vi "Measurement Logic.vi"() -> ()   [LabVIEW 2021, in "PSRR_PMIC.lvlib"]
uses:
  PSRR_PMIC.lvlib
  Measurement Results.ctl
  <instrlib>/niDCPower/nidcpower.llb/niDCPower Get Channel Name From String.vi
  <instrlib>/niDCPower/nidcpower.llb/niDCPower Source Mode.ctl
  <instrlib>/niDCPower/nidcpower.llb/niDCPower Output Function.ctl
  <instrlib>/niDCPower/nidcpower.llb/niDCPower Sense.ctl
  <instrlib>/niDCPower/nidcpower.llb/niDCPower Wait For Event - Event.ctl
  <instrlib>/niFgen/niFgen.llb/niFgen Output Mode.ctl
  <instrlib>/niScope/Controls/niScope vertical coupling.ctl
  <instrlib>/niScope/Controls/niScope trigger slope.ctl
  <instrlib>/niScope/Controls/niScope trigger coupling.ctl
  <instrlib>/niScope/Controls/niScope trigger source.ctl
  <instrlib>/niScope/Utility/niScope Get Channel Name From String.vi
  <instrlib>/niScope/Configure/Trigger/niScope Configure Trigger Edge.vi
  <vilib>/Plug-In SDKs/Measurements/Measure Call Context/Measure Call Context.lvclass
  Measurement Configuration.ctl
panel:
  out "measurement results":T1
  in  "measurement configuration":T2={"DUT setup time"=1.0, "Source resource name"="", "Source current limit"=0.15, "Source voltage level"=10.0, "Load resource name"="", "Load voltage limit range"=6.0, "Load current level"=0.025, "Fgen resource name"="", "Fgen channel name"="", "Fgen pk-pk amplitude"=1.0, "Fgen load impedance"=10000.0, "Fgen start frequency"=10.0, "Fgen stop frequency"=10000000.0, "Fgen frequency sweep points/points per decade"=10, "Fgen sweep type"="Logarithmic", "Fgen standard Waveform"=enum."Sine", "Scope resource name"="", "Scope input channel name"="", "Scope output channel name"="", "Scope probe attenuation"=1.0, "Scope samples per cycle"=1000, "Scope cycles to average"=4} {"Fgen start frequency" format="%#_6p"; "Fgen load impedance" format="%#_6p"; "Fgen pk-pk amplitude" format="%#_6p"}
  out "measure call context out":refnum<class "Measure Call Context.lvclass">
  in  "measure call context in":refnum<class "Measure Call Context.lvclass">
  out "error out":errorcluster
  in  "error in":errorcluster
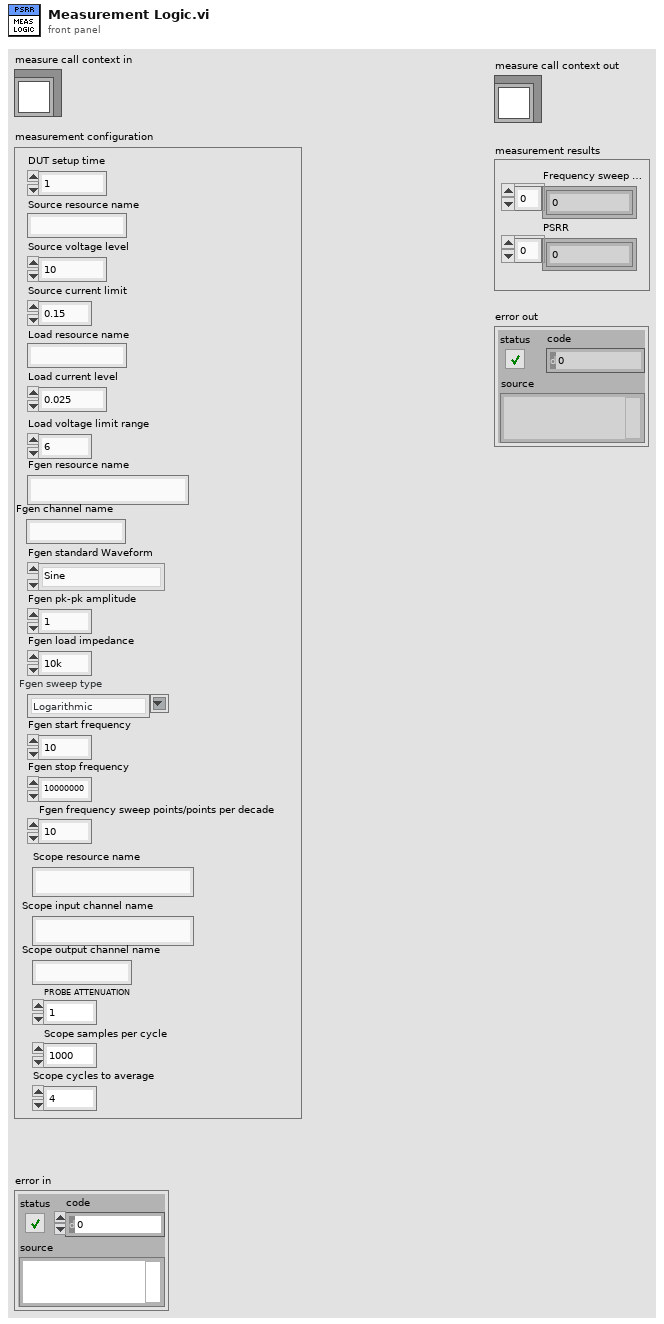
[diagram p1: front panel]
types:
  T1 = typedef "PSRR_PMIC.lvlib/Measurement Results.ctl" = cluster{"Frequency sweep points":dbl[], "PSRR":dbl[]}
  T2 = typedef "PSRR_PMIC.lvlib/Measurement Configuration.ctl" = cluster{"DUT setup time":dbl, "Source resource name":string, "Source current limit":dbl, "Source voltage level":dbl, "Load resource name":string, "Load voltage limit range":dbl, "Load current level":dbl, "Fgen resource name":string, "Fgen channel name":string, "Fgen pk-pk amplitude":dbl, "Fgen load impedance":dbl, "Fgen start frequency":dbl, "Fgen stop frequency":dbl, "Fgen frequency sweep points/points per decade":i32, "Fgen sweep type":string, "Fgen standard Waveform":enum32{"Sine", "Square", "Triangle", "Ramp Up", "Ramp Down", "DC", "Noise"}, "Scope resource name":string, "Scope input channel name":string, "Scope output channel name":string, "Scope probe attenuation":dbl, "Scope samples per cycle":i32, "Scope cycles to average":i32}
  T3 = typedef "niScope trigger coupling.ctl" = u16
  T4 = typedef "niScope trigger slope.ctl" = i32
  T5 = typedef "niScope vertical coupling.ctl" = i32
  T6 = typedef "niFgen Output Mode.ctl" = u32
  T7 = typedef "niDCPower Output Function.ctl" = i32
  T8 = typedef "niDCPower Source Mode.ctl" = i32
  T9 = typedef "niDCPower Wait For Event - Event.ctl" = i32
  T10 = typedef "niDCPower Sense.ctl" = i32
  T11 = enum32{"Sine", "Square", "Triangle", "Ramp Up", "Ramp Down", "DC", "Noise"}
  T12 = typedef "niScope trigger source.ctl" = string
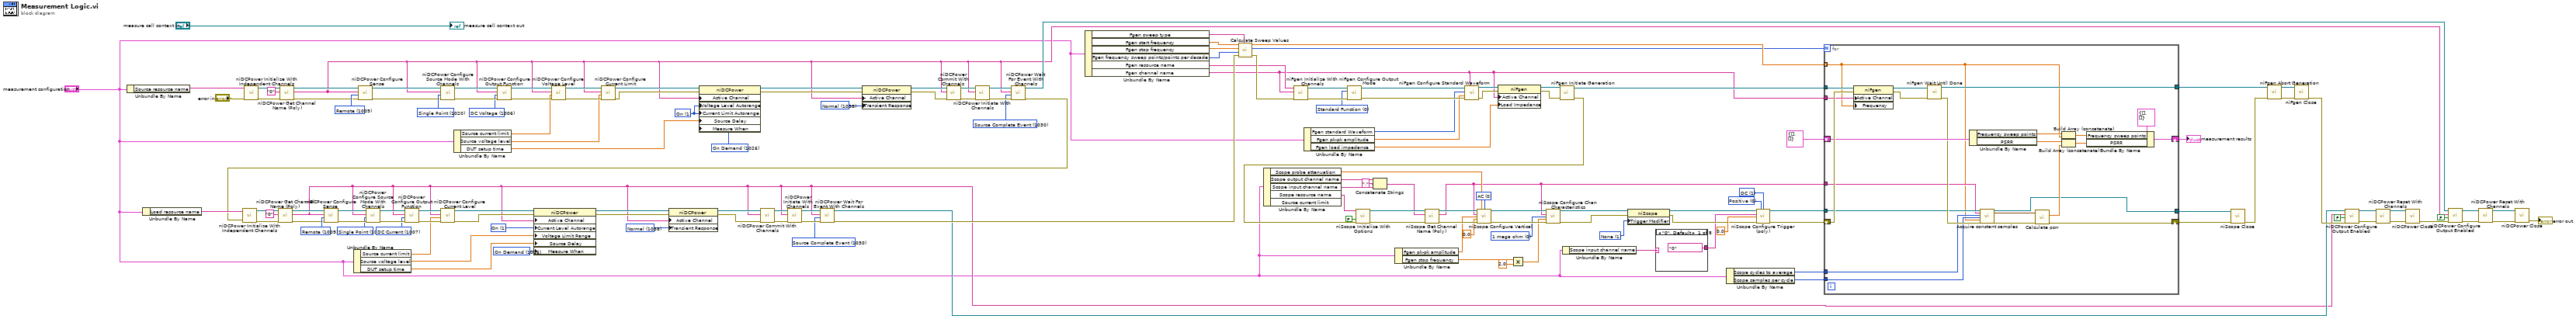
[diagram p0: block diagram]
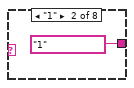
[diagram p2: hidden frame]
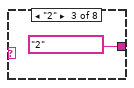
[diagram p3: hidden frame]
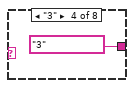
[diagram p4: hidden frame]
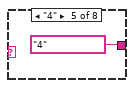
[diagram p5: hidden frame]
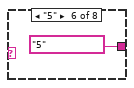
[diagram p6: hidden frame]
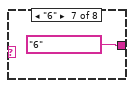
[diagram p7: hidden frame]
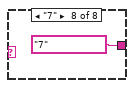
[diagram p8: hidden frame]
diagram:
  w51 = 1 items=["None"=1, "Auto Trigger"=2] ("Triggering:Trigger Modifier")
  w57 = T3 1 items=["AC"=0, "DC"=1, "HF Reject"=3, "LF Reject"=4, "AC Plus HF Reject"=1001] ("trigger coupling")
  w58 = T4 0 items=["Positive", "Negative"] ("trigger slope")
  w60 = T5 0 items=["AC", "DC", "Ground"] ("vertical coupling")
  w63 = u32 0 items=["1 mega ohm"=0, "50 ohms"=2] ("input impedance")
  w79 = T6 0 items=["Standard Function", "Frequency List", "Arbitrary Waveform", "Arbitrary Sequence", "Script"] ("Output Mode (default: 0=Standard Function)")
  w98 = T7 1007 items=["DC Voltage"=1006, "DC Current"=1007, "Pulse Voltage"=1049, "Pulse Current"=1050] ("output function")
  w99 = T8 1020 items=["Single Point"=1020, "Sequence"=1021] ("source mode")
  w24 = 1026 items=["Automatically after Source Complete"=1025, "On Demand"=1026, "On Measure Trigger"=1027] ("Measurement:Advanced:Measure When")
  w101 = 1 items=["Off", "On"] ("Source:DC Current:Current Level Autorange")
  w113 = 1038 items=["Slow"=1041, "Normal"=1038, "Fast"=1039, "Custom"=1042] ("Source:Transient Response")
  w116 = T9 1030 items=["Source Complete Event"=1030, "Measure Complete Event"=1031, "Sequence Iteration Complete Event"=1032, "Sequence Engine Done Event"=1033, "Pulse Complete Event"=1051, "Ready For Pulse Trigger Event"=1052] ("event")
  w119 = T10 1009 items=["Local"=1008, "Remote"=1009] ("sense")
  w122 = T9 1030 items=["Source Complete Event"=1030, "Measure Complete Event"=1031, "Sequence Iteration Complete Event"=1032, "Sequence Engine Done Event"=1033, "Pulse Complete Event"=1051, "Ready For Pulse Trigger Event"=1052] ("event")
  w130 = 1038 items=["Slow"=1041, "Normal"=1038, "Fast"=1039, "Custom"=1042] ("Source:Transient Response")
  w137 = T10 1009 items=["Local"=1008, "Remote"=1009] ("sense")
  w138 = 1026 items=["Automatically after Source Complete"=1025, "On Demand"=1026, "On Measure Trigger"=1027] ("Measurement:Advanced:Measure When")
  w144 = 1 items=["Off", "On"] ("Source:DC Voltage:Current Limit Autorange")
  w146 = T7 1006 items=["DC Voltage"=1006, "DC Current"=1007, "Pulse Voltage"=1049, "Pulse Current"=1050] ("output function")
  w149 = T8 1020 items=["Single Point"=1020, "Sequence"=1021] ("source mode")
  n1 = Unbundle By Name("measurement configuration") -> ("Source resource name"=w150:string)
  n2 = Unbundle By Name("measurement configuration") -> ("Load resource name"=w89:string)
  n3 = call <instrlib>:"niDCPower Initialize With Independent Channels.vi"("error in (no error)"="error in", "resource name"=w150) -> ("error out"=w152:errorcluster, "instrument handle out"=w153:refnum<k15>)  [unwired: 8 in]
  n4 = call-poly <instrlib>:"niDCPower Get Channel Name (Poly).vi"("error in (no error)"=w152, "index"="0", "instrument handle"=w153) -> ("error out"=w120:errorcluster, "name"=w8:string, "instrument handle out"=w121:refnum<k15>)  [unwired: 6 in]
  n5 = Unbundle By Name("measurement configuration") -> ("Source current limit"=w100:dbl, "Source voltage level"=w95:dbl, "DUT setup time"=w110:dbl)
  n6 = call <instrlib>:"niDCPower Configure Sense.vi"("error in (no error)"=w120, "sense"=w137, "channel name"=w8, "instrument handle"=w121) -> ("error out"=w129:errorcluster, "instrument handle out"=w128:refnum<k15>)  [unwired: 6 in]
  n7 = call <instrlib>:"niDCPower Configure Source Mode With Channels.vi"("error in (no error)"=w129, "source mode"=w149, "channel name"=w8, "instrument handle"=w128) -> ("error out"=w148:errorcluster, "instrument handle out"=w147:refnum<k15>)  [unwired: 6 in]
  n8 = Unbundle By Name("measurement configuration") -> ("Source current limit"=w126:dbl, "Source voltage level"=w127:dbl, "DUT setup time"=w125:dbl)
  n9 = call <instrlib>:"niDCPower Configure Output Function.vi"("error in (no error)"=w148, "output function"=w146, "channel name"=w8, "instrument handle"=w147) -> ("error out"=w142:errorcluster, "instrument handle out"=w141:refnum<k15>)  [unwired: 6 in]
  n10 = call <instrlib>:"niDCPower Configure Voltage Level.vi"("error in (no error)"=w142, "voltage level"=w126, "channel name"=w8, "instrument handle"=w141) -> ("error out"=w139:errorcluster, "instrument handle out"=w140:refnum<k15>)  [unwired: 6 in]
  n11 = call <instrlib>:"niDCPower Configure Current Limit.vi"("error in (no error)"=w139, "current limit"=w127, "channel name"=w8, "instrument handle"=w140) -> ("error out"=w145:errorcluster, "instrument handle out"=w143:refnum<k15>)  [unwired: 6 in]
  n12 = property class="niDCPower"(reference=w143, error in=w145, "Active Channel"=w8, "Voltage Level Autorange"=w144, "Current Limit Autorange"=w144, "Source Delay"=w125, "Measure When"=w138) -> (reference out=w134:refnum<k15>, error out=w133:errorcluster)
  n13 = property class="niDCPower"(reference=w134, error in=w133, "Active Channel"=w8, "Transient Response"=w130) -> (reference out=w132:refnum<k15>, error out=w131:errorcluster)
  n14 = call <instrlib>:"niDCPower Commit With Channels.vi"("error in (no error)"=w131, "channel name"=w8, "instrument handle"=w132) -> ("error out"=w135:errorcluster, "instrument handle out"=w136:refnum<k15>)  [unwired: 7 in]
  n15 = call <instrlib>:"niDCPower Initiate With Channels.vi"("error in (no error)"=w135, "channel name"=w8, "instrument handle"=w136) -> ("error out"=w123:errorcluster, "instrument handle out"=w124:refnum<k15>)  [unwired: 7 in]
  n16 = call <instrlib>:"niDCPower Wait For Event With Channels.vi"("error in (no error)"=w123, "event"=w122, "channel name"=w8, "instrument handle"=w124) -> ("error out"=w70:errorcluster, "instrument handle out"=w11:refnum<k15>)  [unwired: 6 in]
  n17 = call <instrlib>:"niDCPower Initialize With Independent Channels.vi"("error in (no error)"=w70, "resource name"=w89) -> ("error out"=w93:errorcluster, "instrument handle out"=w94:refnum<k15>)  [unwired: 8 in]
  n18 = call-poly <instrlib>:"niDCPower Get Channel Name (Poly).vi"("error in (no error)"=w93, "index"="0", "instrument handle"=w94) -> ("error out"=w90:errorcluster, "name"=w9:string, "instrument handle out"=w91:refnum<k15>)  [unwired: 6 in]
  n19 = call <instrlib>:"niDCPower Configure Sense.vi"("error in (no error)"=w90, "sense"=w119, "channel name"=w9, "instrument handle"=w91) -> ("error out"=w104:errorcluster, "instrument handle out"=w107:refnum<k15>)  [unwired: 6 in]
  n20 = call <instrlib>:"niDCPower Configure Source Mode With Channels.vi"("error in (no error)"=w104, "source mode"=w99, "channel name"=w9, "instrument handle"=w107) -> ("error out"=w103:errorcluster, "instrument handle out"=w106:refnum<k15>)  [unwired: 6 in]
  n21 = call <instrlib>:"niDCPower Configure Output Function.vi"("error in (no error)"=w103, "output function"=w98, "channel name"=w9, "instrument handle"=w106) -> ("error out"=w102:errorcluster, "instrument handle out"=w105:refnum<k15>)  [unwired: 6 in]
  n22 = call <instrlib>:"niDCPower Configure Current Level.vi"("error in (no error)"=w102, "current level"=w100, "channel name"=w9, "instrument handle"=w105) -> ("error out"=w96:errorcluster, "instrument handle out"=w97:refnum<k15>)  [unwired: 6 in]
  n23 = property class="niDCPower"(reference=w97, error in=w96, "Active Channel"=w9, "Current Level Autorange"=w101, "Voltage Limit Range"=w95, "Source Delay"=w110, "Measure When"=w24) -> (reference out=w112:refnum<k15>, error out=w111:errorcluster)
  n24 = property class="niDCPower"(reference=w112, error in=w111, "Active Channel"=w9, "Transient Response"=w113) -> (reference out=w109:refnum<k15>, error out=w108:errorcluster)
  n25 = call <instrlib>:"niDCPower Commit With Channels.vi"("error in (no error)"=w108, "channel name"=w9, "instrument handle"=w109) -> ("error out"=w114:errorcluster, "instrument handle out"=w115:refnum<k15>)  [unwired: 7 in]
  n26 = call <instrlib>:"niDCPower Initiate With Channels.vi"("error in (no error)"=w114, "channel name"=w9, "instrument handle"=w115) -> ("error out"=w118:errorcluster, "instrument handle out"=w117:refnum<k15>)  [unwired: 7 in]
  n27 = call <instrlib>:"niDCPower Wait For Event With Channels.vi"("error in (no error)"=w118, "event"=w116, "channel name"=w9, "instrument handle"=w117) -> ("error out"=w77:errorcluster, "instrument handle out"=w10:refnum<k15>)  [unwired: 6 in]
  n28 = Unbundle By Name("measurement configuration") -> ("Fgen sweep type"=w76:string, "Fgen start frequency"=w25:dbl, "Fgen stop frequency"=w75:dbl, "Fgen frequency sweep points/points per decade"=w74:i32, "Fgen resource name"=w6:string, "Fgen channel name"=w5:string)
  n29 = call "Calculate Sweep Values.vi"("Sweep type"=w76, "error in"=w77, "Points"=w74, "Stop level"=w75, "Start level"=w25) -> ("error out"=w78:errorcluster, "Sweep points"=w28:i32, "Sweep values"=w29:dbl[])  [unwired: 4 in]
  n30 = Unbundle By Name("measurement configuration") -> ("Scope probe attenuation"=w46:dbl, "Scope output channel name"=w43:string, "Scope input channel name"=w45:string, "Scope resource name"=w59:string)  [unwired: 1 out]
  n31 = call <instrlib>:"niFgen Initialize With Channels.vi"("error in (no error)"=w78, "Channel Name"=w5, "Resource Name"=w6) -> ("error out"=w84:errorcluster, "Instrument Handle Out"=w87:refnum<k15>)  [unwired: 7 in]
  n32 = Unbundle By Name("measurement configuration") -> ("Fgen standard Waveform"=w72:T11, "Fgen pk-pk amplitude"=w71:dbl, "Fgen load impedance"=w73:dbl)
  n33 = call <instrlib>:"niFgen Configure Output Mode.vi"("error in (no error)"=w84, "Output Mode (default: 0=Standard Function)"=w79, "Instrument Handle"=w87) -> ("error out"=w83:errorcluster, "Instrument Handle Out"=w86:refnum<k15>)  [unwired: 6 in]
  n34 = Concatenate Strings(w43, "," ("string"), w45) -> (w42:string)
  n35 = Unbundle By Name("measurement configuration") -> ("Fgen pk-pk amplitude"=w4:dbl, "Fgen stop frequency"=w49:dbl)
  n36 = call <instrlib>:"niFgen Configure Standard Waveform.vi"("Instrument Handle"=w86, "Channel Name"=w5, "Waveform"=w72, "Amplitude"=w71, "error in (no error)"=w83) -> ("Instrument Handle Out"=w85:refnum<k15>, "error out"=w82:errorcluster)  [unwired: 9 in]
  n37 = property class="niFgen"(reference=w85, error in=w82, "Active Channel"=w5, "Load Impedance"=w73) -> (reference out=w81:refnum<k15>, error out=w80:errorcluster)
  n38 = Multiply(x=w49, y=2.0) -> (x*y=w50:dbl)
  n39 = call <instrlib>:"niFgen Initiate Generation.vi"("error in (no error)"=w80, "Instrument Handle"=w81) -> ("error out"=w47:errorcluster, "Instrument Handle Out"=w30:refnum<k15>)  [unwired: 8 in]
  n40 = call <instrlib>:"niScope Initialize With Options.vi"("resource name"=w59, "reset device"=FALSE, "error in"=w47) -> ("instrument handle"=w69:refnum<k15>, "error out"=w66:errorcluster)  [unwired: 11 in]
  n41 = call-poly <instrlib>:"niScope Get Channel Name (Poly).vi"("instrument handle"=w69, "index"=w42, "error in"=w66) -> ("instrument handle out"=w68:refnum<k15>, "channel name"=w31:string, "error out"=w65:errorcluster)  [unwired: 10 in]
  n42 = call <instrlib>:"niScope Configure Vertical.vi"("instrument handle"=w68, "probe attenuation"=w46, "vertical coupling"=w60, "channels"=w31, "vertical range"=w4, "vertical offset"=0.0, "error in"=w65) -> ("instrument handle out"=w67:refnum<k15>, "error out"=w64:errorcluster)  [unwired: 7 in]
  n43 = call <instrlib>:"niScope Configure Chan Characteristics.vi"("instrument handle"=w67, "channels"=w31, "input impedance"=w63, "maximum input frequency"=w50, "error in"=w64) -> ("instrument handle out"=w55:refnum<k15>, "error out"=w54:errorcluster)  [unwired: 9 in]
  n44 = Unbundle By Name("measurement configuration") -> ("Scope input channel name"=w1:string)
  n45 = property on="Property Node" class="niScope"(reference=w55, error in=w54, "Trigger Modifier"=w51) -> (reference out=w53:refnum<k15>, error out=w52:errorcluster)
  n46 = case shown="\"0\", Default" w1 {
    tunnel: [T12 "0" ("trigger source") T12 "1" ("trigger source") T12 "2" ("trigger source") T12 "3" ("trigger source") T12 "4" ("trigger source") T12 "5" ("trigger source") T12 "6" ("trigger source") T12 "7" ("trigger source")] -> w2
    frame "0", Default {
    }
    frame "1" {
    }
    frame "2" {
    }
    frame "3" {
    }
    frame "4" {
    }
    frame "5" {
    }
    frame "6" {
    }
    frame "7" {
    }
  }
  n47 = Unbundle By Name("measurement configuration") -> ("Scope cycles to average"=w41:i32, "Scope samples per cycle"=w40:i32)
  n48 = call-poly <instrlib>:"niScope Configure Trigger (poly).vi"("instrument handle"=w53, "trigger slope"=w58, "trigger coupling"=w57, "trigger source"=w2, "trigger level"=0.0, "error in"=w52) -> ("instrument handle out"=w32:refnum<k15>, "error out"=w33:errorcluster)  [unwired: 8 in]
  n49 = for {
    N: w28 -> [_]
    tunnel: w30 -> [w184]
    tunnel: w41 -> [w165]
    tunnel: w40 -> [w164]
    tunnel: w31 -> [w166]
    tunnel: w29 -> [w163] mode=indexing
    shift-right: [w172] -> w35
    shift-left: w33 -> [w183]
    tunnel: [w182] -> w36
    tunnel: [w168] -> w34
    tunnel: w32 -> [w167]
    shift-right: [w180] -> w27
    shift-left: T1 {"Frequency sweep points"=[], "PSRR"=[]} ("Measurement Results") -> [w179]
    tunnel: w5 -> [w174]
    n50 = property class="niFgen"(reference=w184, error in=w183, "Active Channel"=w174, "Frequency"=w163) -> (reference out=w185:refnum<k15>, error out=w186:errorcluster)
    n51 = call <instrlib>:"niFgen Wait Until Done.vi"("error in (no error)"=w186, "Instrument Handle"=w185) -> ("error out"=w171:errorcluster, "Instrument Handle Out"=w182:refnum<k15>)  [unwired: 8 in]
    n52 = Unbundle By Name(w179) -> ("Frequency sweep points"=w178:dbl[], "PSRR"=w177:dbl[])
    n53 = call "Acquire constant samples.vi"("Instrument handle"=w167, "Channel(s)"=w166, "Cycles to acquire"=w165, "Samples/cycle"=w164, "Frequency"=w163, "error in (no error)"=w171) -> ("Instrument handle out"=w168:refnum<k15>, "Waveform(s)"=w169:waveform(dbl)[], "error out"=w170:errorcluster)  [unwired: 11 in]
    n54 = call "Calculate psrr.vi"("error in (no error)"=w170, "Time signal(s) in"=w169) -> ("error out"=w172:errorcluster, "PSRR"=w173:dbl)  [unwired: 8 in]
    n55 = Build Array (concatenate)(w178, w163) -> (w176:dbl[])
    n56 = Build Array (concatenate)(w177, w173) -> (w175:dbl[])
    n57 = Bundle By Name(cluster=T1 {"Frequency sweep points"=[], "PSRR"=[]} ("Measurement Results"), "Frequency sweep points"=w176, "PSRR"=w175) -> (w180:T1)
  }
  "measurement results" <- w27
  n58 = call <instrlib>:"niScope Close.vi"("instrument handle"=w34, "error in"=w35) -> ("error out"=w39:errorcluster)  [unwired: 13 in]
  n59 = call <instrlib>:"niFgen Abort Generation.vi"("error in (no error)"=w39, "Instrument Handle"=w36) -> ("error out"=w38:errorcluster, "Instrument Handle Out"=w37:refnum<k15>)  [unwired: 8 in]
  n60 = call <instrlib>:"niFgen Close.vi"("error in (no error)"=w38, "Instrument Handle"=w37) -> ("error out"=w12:errorcluster)  [unwired: 9 in]
  n61 = call <instrlib>:"niDCPower Configure Output Enabled.vi"("error in (no error)"=w12, "output enabled"=FALSE, "channel name"=w9, "instrument handle"=w10) -> ("error out"=w17:errorcluster, "instrument handle out"=w16:refnum<k15>)  [unwired: 6 in]
  n62 = call <instrlib>:"niDCPower Reset With Channels.vi"("error in (no error)"=w17, "instrument handle"=w16) -> ("error out"=w14:errorcluster, "instrument handle out"=w15:refnum<k15>)  [unwired: 8 in]
  n63 = call <instrlib>:"niDCPower Close.vi"("error in (no error)"=w14, "instrument handle"=w15) -> ("error out"=w18:errorcluster)  [unwired: 9 in]
  n64 = call <instrlib>:"niDCPower Configure Output Enabled.vi"("error in (no error)"=w18, "output enabled"=FALSE, "channel name"=w8, "instrument handle"=w11) -> ("error out"=w19:errorcluster, "instrument handle out"=w20:refnum<k15>)  [unwired: 6 in]
  n65 = call <instrlib>:"niDCPower Reset With Channels.vi"("error in (no error)"=w19, "instrument handle"=w20) -> ("error out"=w22:errorcluster, "instrument handle out"=w23:refnum<k15>)  [unwired: 8 in]
  n66 = call <instrlib>:"niDCPower Close.vi"("error in (no error)"=w22, "instrument handle"=w23) -> ("error out"=→"error out":errorcluster)  [unwired: 9 in]
  "measure call context out" <- "measure call context in"
